vi "AIO.vi"() -> ()   [LabVIEW 2016]
uses:
  <vilib>/rvi/Emulation/niFpgaGetClockAttributes.vi
  <vilib>/rvi/Emulation/niFpgaSctlEmulationGetInTimedLoop.vi
  <vilib>/rvi/Emulation/niFpgaEmulationReportErrorSimple.vi
  <vilib>/rvi/eio/common/nirviEmuTemplateMethod_errors.vi
  <vilib>/rvi/Emulation/niFpgaCriticalErrorInLSC.vi
  <vilib>/eio/EIONode/EIONode.xnode
panel:
  out "ConnectorC/AI0":i16
  in  "ConnectorC/AO0":i16
  out "ConnectorB/AI2":u16
  out "ConnectorB/AI1":u16
  out "ConnectorB/AI0":u16
  in  "stop":bool
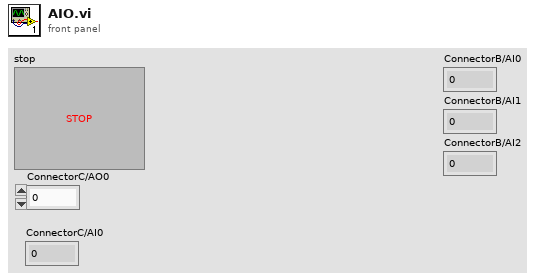
[diagram p1: front panel]
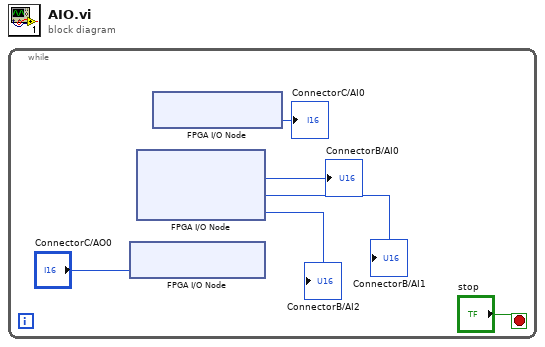
[diagram p0: block diagram]
diagram:
  n1 = while {
    stop <- "stop" stop-if-true
    n2 = xnode "FPGA I/O Node"("ConnectorC/AO0"="ConnectorC/AO0") -> ()  [unwired: 1 in, 1 out]
    n3 = xnode "FPGA I/O Node"() -> ("ConnectorB/AI0"=→"ConnectorB/AI0":u16, "ConnectorB/AI1"=→"ConnectorB/AI1":u16, "ConnectorB/AI2"=→"ConnectorB/AI2":u16)  [unwired: 3 in, 3 out]
    n4 = xnode "FPGA I/O Node"() -> ("ConnectorC/AI0"=→"ConnectorC/AI0":i16)  [unwired: 1 in, 1 out]
  }
